vi "Memory.Pointer.Internal.Duplicate2.vi"(8 "error in (no error)":errorcluster, 11 "pointer in":refnum<class "Memory.Pointer.Internal.lvclass">) -> (0 "error out":errorcluster, 2 "new pointer":refnum<class "Memory.Pointer.Internal.lvclass">, 3 "pointer out":refnum<class "Memory.Pointer.Internal.lvclass">)   [LabVIEW 2016]
doc: "Allocates a <b>new pointer</b> with a copy of the data referenced by the provided <b>pointer</b>."
uses:
  Internal/Memory.Pointer.Internal.lvclass
  Memory.Pointer.lvclass
  Memory.Pointer.Copy All.Safe.vi
  C:/Git/SourceTree/DSF/Source/Submodules/Memory/Source/Classes/Pointer/Memory.Pointer.lvclass
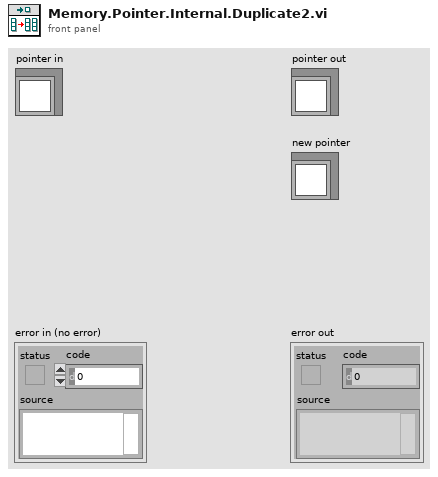
[diagram p1: front panel]
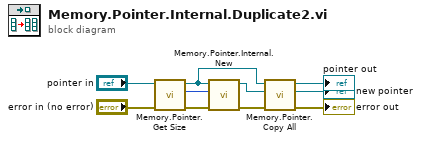
[diagram p0: block diagram]
diagram:
  n1 = call "Memory.Pointer.Get Size.vi"("Pointer in"="pointer in") -> ("size"=w3:u64, "Pointer out"=w1:refnum<class "Memory.Pointer.Internal.lvclass">)  [unwired: 9 in]
  n2 = call "Memory.Pointer.Internal.New.vi"("error in (no error)"="error in (no error)", "size"=w3, "Pointer type-specifier"=w1) -> ("error out"=w7:errorcluster, "pointer"=w2:refnum<class "Memory.Pointer.Internal.lvclass">)  [unwired: 7 in]
  n3 = call-poly "Memory.Pointer.Copy All.vi"("error in (no error)"=w7, "dst pointer in"=w2, "src pointer in"=w1) -> ("error out"=→"error out":errorcluster, "dst pointer out"=→"new pointer":refnum<class "Memory.Pointer.Internal.lvclass">, "src pointer out"=→"pointer out":refnum<class "Memory.Pointer.Internal.lvclass">)  [unwired: 6 in]
